vi "АЛУ.vi"(2 "B":T4, 3 "A":T5, 4 "ClearAcc":bool, 5 "Exec":bool, 6 "c":bool, 7 "Func":T3) -> (0 "Flags":T1, 1 "R":T2)   [LabVIEW 2013]
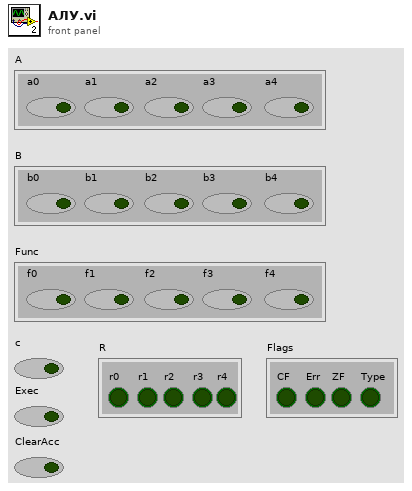
[diagram p1: front panel]
types:
  T1 = cluster{"CF":bool, "Err":bool, "ZF":bool, "Type":bool}
  T2 = cluster{"r0":bool, "r1":bool, "r2":bool, "r3":bool, "r4":bool}
  T3 = cluster{"f0":bool, "f1":bool, "f2":bool, "f3":bool, "f4":bool}
  T4 = cluster{"b0":bool, "b1":bool, "b2":bool, "b3":bool, "b4":bool}
  T5 = cluster{"a0":bool, "a1":bool, "a2":bool, "a3":bool, "a4":bool}
  T6 = cluster{"q4":bool, "q3":bool, "q2":bool, "q1":bool, "q0":bool}
  T7 = cluster{"CF":bool, "Err":bool, "ZF":bool, "Type":bool, bool}
  T8 = cluster{"q4":bool, "q3":bool, "q2":bool, "q1":bool}
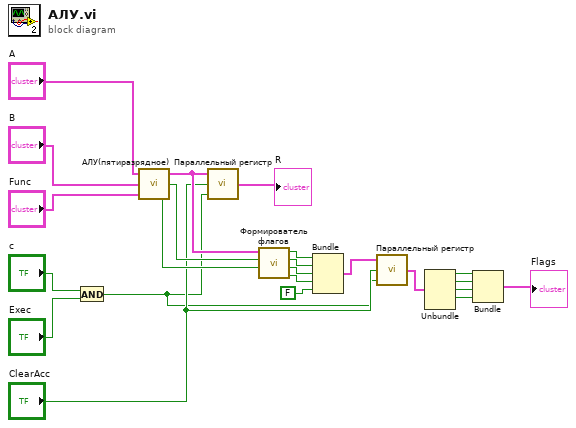
[diagram p0: block diagram]
diagram:
  n1 = And(x="c", y="Exec") -> (x .and. y?=w7:bool)
  n2 = call "АЛУ(пятиразрядное).vi"("Func"="Func", "B"="B", "A"="A") -> ("Type"=w15:bool, "s1"=w16:bool, "R"=w17:T2)
  n3 = call "Параллельный регистр.vi"("C"=w7, "Reset"="ClearAcc", "Cluster"=w17) -> ("output cluster"=→"R":T6)
  n4 = call "Формирователь флагов.vi"("Type"=w15, "s1"=w16, "R"=w17) -> ("Type"=w10:bool, "ZF"=w12:bool, "Err"=w13:bool, "CF"=w14:bool)  [unwired: 1 in]
  n5 = Bundle("CF"=w14, "Err"=w13, "ZF"=w12, "Type"=w10, FALSE) -> (w11:T7)  [unwired: 1 in]
  n6 = call "Параллельный регистр.vi"("C"=w7, "Reset"="ClearAcc", "Cluster"=w11) -> ("output cluster"=w6:T6)
  n7 = Unbundle(w6) -> ("q4"=w5:bool, "q3"=w3:bool, "q2"=w2:bool, "q1"=w1:bool)  [unwired: 1 out]
  n8 = Bundle("q4"=w5, "q3"=w3, "q2"=w2, "q1"=w1) -> (→"Flags":T8)  [unwired: 1 in]
